vi "sv_Peak Weighting (1 Ch).vi"(4 "error IO":errorcluster, 5 "spectrum info in":T1 {"x-axis units" items=["Time (s)"=0, "Frequency-CB (Hz)"=1, "Frequency-CPB (Hz)"=1248, "Frequency-Arbitrary (Hz)"=2357, "Quefrency (s)"=2, "Revolutions (rev)"=3, "Order"=4, "Speed (RPM)"=11, "Speed (rad/s)"=21, "Index"=65535]; "weighting filter" items=["Linear", "A-weighting", "B-weighting", "C-weighting", "ITU-R 468-4", "Dolby", "CCITT", "C-message", "Wb", "Wc", "Wd", "We", "Wf", "Wh", "Wj", "Wk", "Wm", "AES17 20 kHz lowpass", "AES17 40 kHz lowpass", "AES17 20 kHz highpass", "AES17 40 kHz highpass"]; "dB reference [EU]" format="%.2f"; "engineering units" items=["custom..."=0, "V"=1, "A"=21, "C"=30, "pC"=31, "s"=32, "-"=29, "Pa"=2, "N"=20, "g"=3, "m/s^2"=4, "m/s"=5, "m"=6, "mm/s"=12, "mm"=13, "micron/s"=14, "micron"=15, "in/s^2"=7, "in/s"=8, "in"=9, "mil/s"=10, "mil"=11, "rad/s^2"=16, "rad/s"=17, "rad"=18, "deg/s^2"=26, "deg/s"=27, "deg"=28, "RPM"=22, "cycle/s^2"=23, "Hz"=24, "cycle"=25, "strain"=19]; "spectral info"."window" items=["None "=0, "Hanning"=1, "Hamming"=2, "Blackman-Harris"=3, "Exact Blackman"=4, "Blackman"=5, "Flat Top"=6, "4 Term B-Harris "=7, "7 Term B-Harris"=8, "Low Sidelobe"=9, "Force - Exponential"=10, "Gaussian"=62]}, 6 "weighting":u16, 7 "peaks":cluster{"freq. or order":dbl, "value":dbl}[](array[cluster])) -> (0 "error out":errorcluster, 1 "spectrum info out":T1 {"x-axis units" items=["Time (s)"=0, "Frequency-CB (Hz)"=1, "Frequency-CPB (Hz)"=1248, "Frequency-Arbitrary (Hz)"=2357, "Quefrency (s)"=2, "Revolutions (rev)"=3, "Order"=4, "Speed (RPM)"=11, "Speed (rad/s)"=21, "Index"=65535]; "weighting filter" items=["Linear", "A-weighting", "B-weighting", "C-weighting", "ITU-R 468-4", "Dolby", "CCITT", "C-message", "Wb", "Wc", "Wd", "We", "Wf", "Wh", "Wj", "Wk", "Wm", "AES17 20 kHz lowpass", "AES17 40 kHz lowpass", "AES17 20 kHz highpass", "AES17 40 kHz highpass"]; "dB reference [EU]" format="%.2f"; "engineering units" items=["custom..."=0, "V"=1, "A"=21, "C"=30, "pC"=31, "s"=32, "-"=29, "Pa"=2, "N"=20, "g"=3, "m/s^2"=4, "m/s"=5, "m"=6, "mm/s"=12, "mm"=13, "micron/s"=14, "micron"=15, "in/s^2"=7, "in/s"=8, "in"=9, "mil/s"=10, "mil"=11, "rad/s^2"=16, "rad/s"=17, "rad"=18, "deg/s^2"=26, "deg/s"=27, "deg"=28, "RPM"=22, "cycle/s^2"=23, "Hz"=24, "cycle"=25, "strain"=19]; "spectral info"."window" items=["None "=0, "Hanning"=1, "Hamming"=2, "Blackman-Harris"=3, "Exact Blackman"=4, "Blackman"=5, "Flat Top"=6, "4 Term B-Harris "=7, "7 Term B-Harris"=8, "Low Sidelobe"=9, "Force - Exponential"=10, "Gaussian"=62]}, 2 "unit label":string, 3 "weighted peaks":cluster{"freq. or order":dbl, "value":dbl}[](array[cluster]))   [LabVIEW 2017]
uses:
  <vilib>/addons/_NISVFA/_Shared subVIs/Controls/svc_Spectrum Info.ctl
  <vilib>/addons/_NISVFA/_Shared subVIs/Controls/svc_X-Axis Units.ctl
  <vilib>/addons/_NISVFA/_Shared subVIs/Controls/svc_Spectrum Type.ctl
  <vilib>/addons/_NISVFA/_Shared subVIs/Controls/svc_Engineering Units Text Ring.ctl
  <vilib>/addons/_NISVFA/_Shared subVIs/Controls/svc_Weighting Filter Text Ring.ctl
  <vilib>/addons/_NISVFA/_Shared subVIs/Controls/svc_Complimentary Spectrum Units.ctl
  <vilib>/addons/_NISVFA/_Shared subVIs/Common/svc_Get Weighting Enum and Labels.vi
  <vilib>/addons/_NISVFA/_Shared subVIs/Common/svc_Unit Label Lexical Class.vi
  <vilib>/addons/_NISVFA/_Shared subVIs/Common/svc_Engineering Units to Unit Label.vi
  <vilib>/addons/_NISVFA/_Shared subVIs/Common/svc_Format Value (DBL).vi
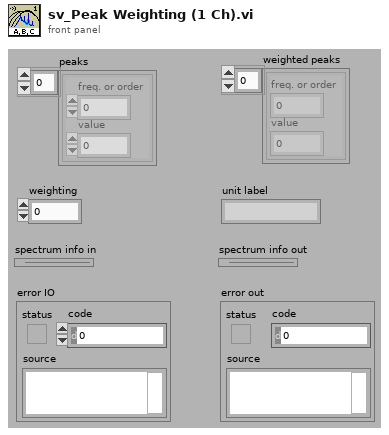
[diagram p1: front panel]
types:
  T1 = typedef "svc_Spectrum Info.ctl" = cluster{"channel name":string, "description":string, "x-axis units":T2, "spectral info":cluster{"spectrum type":T3, "linear/dB":enum16{"linear", "dB"}, "window":u16, "window size":i32, "FFT size":i32}, "engineering units":T4, "custom label":string, "dB reference [EU]":dbl, "peak units":enum16{"rms", "peak", "peak-peak"}, "weighting filter":T5, "spectral density?":bool, "unit label":string, "spectrum skewed?":bool, "complimentary spectrum units":T6}
  T2 = typedef "svc_X-Axis Units.ctl" = u16
  T3 = typedef "svc_Spectrum Type.ctl" = enum16{"FFT Spectrum [complex]", "Amplitude [Magnitude]", "Power [Magnitude^2]", "Cross Spectrum [complex]", "Frequency Response [Complex]"}
  T4 = typedef "svc_Engineering Units Text Ring.ctl" = u16
  T5 = typedef "svc_Weighting Filter Text Ring.ctl" = u16
  T6 = typedef "svc_Complimentary Spectrum Units.ctl" = enum16{"none", "radians", "degrees", "cycles", "imaginary"}
  T7 = enum16{"FFT Spectrum [complex]", "Amplitude [Magnitude]", "Power [Magnitude^2]", "Cross Spectrum [complex]", "Frequency Response [Complex]"}
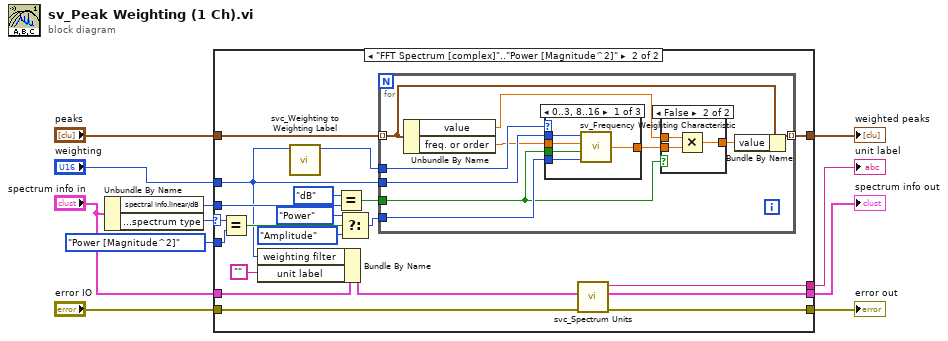
[diagram p0: block diagram]
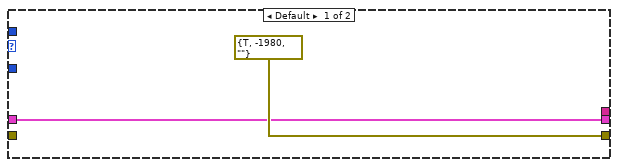
[diagram p2: hidden frame]
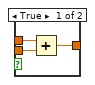
[diagram p3: hidden frame]
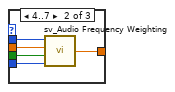
[diagram p4: hidden frame]
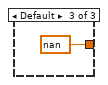
[diagram p5: hidden frame]
diagram:
  n1 = Unbundle By Name("spectrum info in") -> ("spectral info.linear/dB"=w1:enum16{"linear", "dB"}, "spectral info.spectrum type"=w3:T3)
  n2 = case shown="\"FFT Spectrum [complex]\"..\"Power [Magnitude^2]\"" w3 {
    selector: w3 -> [_ w32]
    tunnel: "peaks" -> [_ w23]
    tunnel: "weighting" -> [_ w14]
    tunnel: [errorcluster {"status"=TRUE, "code"=-1980, "source"=""} ("error IO") w18] -> w5
    tunnel: T7."Power [Magnitude^2]" ("y") -> [_ w33]
    tunnel: "error IO" -> [_ w19]
    tunnel: [_ w22] -> w7
    tunnel: w1 -> [_ w27]
    tunnel: "spectrum info in" -> [w12 w21]
    tunnel: [w12 w17] -> w10
    tunnel: [_ w16] -> w6
    frame Default {
    }
    frame "FFT Spectrum [complex]".."Power [Magnitude^2]" {
      n3 = Equal?(x=w32, y=w33) -> (x = y?=w31:bool)
      n4 = Bundle By Name(cluster=w21, "weighting filter"=w14, "unit label"="") -> (w20:T1)
      n5 = call <vilib>:"svc_Weighting to Weighting Label.vi"("weighting filter"=w14) -> ("weighting enum"=w15:T5)  [unwired: 9 in, 1 out]
      n6 = Equal?(x=enum16{"linear", "dB"}."dB" ("y"), y=w27) -> (x = y?=w25:bool)
      n7 = Select(t=enum16{"Power", "Amplitude"}."Power" ("spectrum type"), s=w31, f=enum16{"Power", "Amplitude"}."Amplitude" ("spectrum type")) -> (s? t:f=w30:enum16{"Power", "Amplitude"})
      n8 = for {
        tunnel: [w35] -> w22 mode=indexing
        tunnel: w14 -> [w43]
        tunnel: w30 -> [w42]
        tunnel: w25 -> [w37]
        tunnel: w15 -> [w41]
        tunnel: w23 -> [w36] mode=indexing
        n9 = Unbundle By Name(w36) -> ("value"=w38:dbl, "freq. or order"=w40:dbl)
        n10 = case shown="0..3, 8..16" w41 {
          tunnel: [w54 w55 nan ("relative response level")] -> w39
          tunnel: w40 -> [w53 w58 _]
          tunnel: w43 -> [w52 w59 _]
          tunnel: w42 -> [w51 w56 _]
          tunnel: w37 -> [w50 w57 _]
          frame 0..3, 8..16 {
            n11 = call <vilib>:"sv_Frequency Weighting Characteristic.vi"("spectrum type"=w51, "dB On (T)"=w50, "frequency [Hz]"=w53, "weighting filter"=w52) -> ("relative response level"=w54:dbl)
          }
          frame 4..7 {
            n12 = call <vilib>:"sv_Audio Frequency Weighting.vi"("spectrum type"=w56, "dB On (T)"=w57, "frequency [Hz]"=w58, "weighting filter"=w59) -> ("relative response level"=w55:dbl)
          }
          frame Default {
          }
        }
        n13 = case shown="False" w37 {
          tunnel: w39 -> [w46 w49]
          tunnel: [w45 w48] -> w34
          tunnel: w38 -> [w44 w47]
          frame True {
            n14 = Add(x=w44, y=w46) -> (x+y=w45:dbl)
          }
          frame False {
            n15 = Multiply(x=w47, y=w49) -> (x*y=w48:dbl)
          }
        }
        n16 = Bundle By Name(cluster=w36, "value"=w34) -> (w35:cluster{"freq. or order":dbl, "value":dbl})
      }
      n17 = call <vilib>:"svc_Spectrum Units.vi"("error in (no error)"=w19, "spectrum info in"=w20) -> ("error out"=w18:errorcluster, "spectrum info out"=w17:T1, "unit label"=w16:string)  [unwired: 2 in, 1 out]
    }
  }
  "spectrum info out" <- w10
  "weighted peaks" <- w7
  "unit label" <- w6
  "error out" <- w5
